vi "testMaster.vi"() -> ()   [LabVIEW 2015]
uses:
  support/Slave Device State.ctl
  support/Network Stream Writer.ctl
  NetworkStream/NetworkStreamData.ctl
  <vilib>/dex/Stream Element Allocation Mode.ctl
  <resource>/objmgr/ni.dex.rc
  NetworkStream/NetworkStream.lvlib
panel:
  out "DeviceState":T1
  in  "data":i32
  in  "Message":string
  in  "stop VI":bool
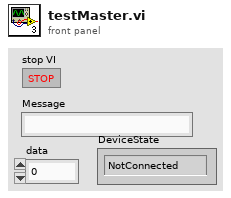
[diagram p1: front panel]
types:
  T1 = typedef "Slave Device State.ctl" = enum16{"NotConnected", "Connected"}
  T2 = typedef "Network Stream Writer.ctl" = cluster{"Hash":u64, "writer endpoint":refnum<k21>, "Sequence Number":u64}
  T3 = typedef "NetworkStream.lvlib/NetworkStreamData.ctl" = cluster{"Command/Status":string, "Data":variant, "Session Hash":u64, "Sequence Number":u64}
  T4 = typedef "Stream Element Allocation Mode.ctl" = u32
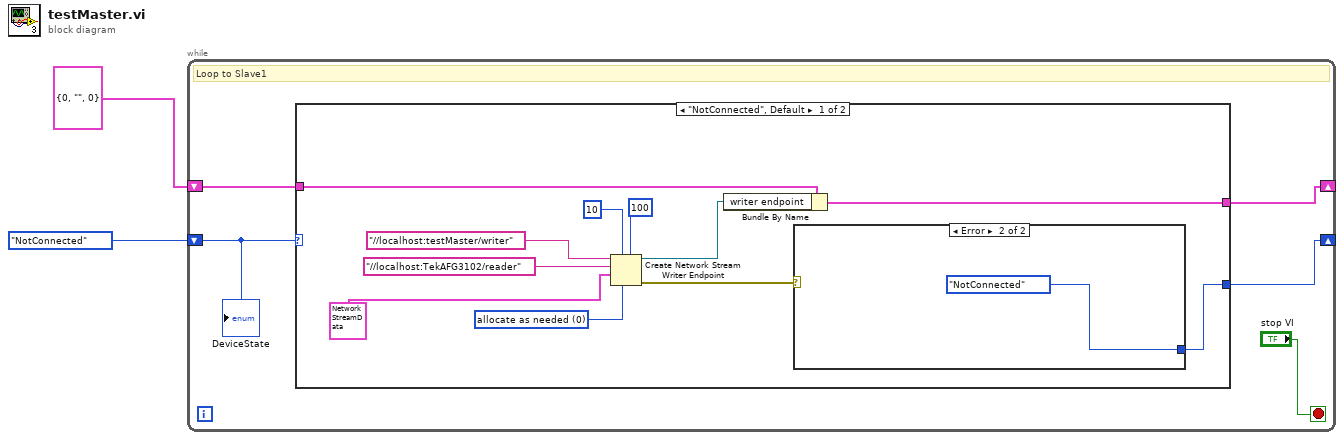
[diagram p0: block diagram]
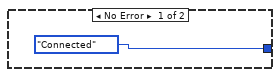
[diagram p2: hidden frame]
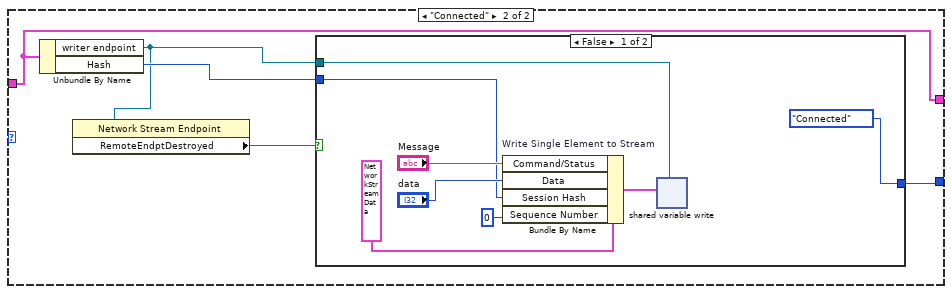
[diagram p3: hidden frame]
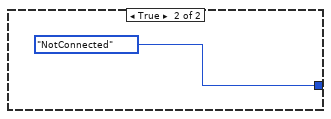
[diagram p4: hidden frame]
diagram:
  n1 = while {
    shift-right: [w5] -> _
    shift-left: T2 {"Hash"=0, "writer endpoint"="", "Sequence Number"=0} ("DeviceData") -> [w6]
    shift-right: [w4] -> _
    shift-left: Slave_Device_State."NotConnected" ("DeviceState") -> [w7]
    stop <- "stop VI" stop-if-true
    # "Loop to Slave1"
    n2 = case shown="\"NotConnected\", Default" w7 {
      tunnel: w6 -> [w18 w24]
      tunnel: [w15 w24] -> w5
      tunnel: [w13 w21] -> w4
      frame "NotConnected", Default {
        w10 = T4 0 items=["allocate as needed", "pre-allocate"] ("element allocation mode")
        n3 = Create Network Stream Writer Endpoint(5:100 ("timeout in ms (-1)"), 6:w10, 7:10 ("writer buffer size"), 9:T3 {"Command/Status"="", "Data"=variant, "Session Hash"=0, "Sequence Number"=0} ("NetworkStreamCluster"), 10:"//localhost:TekAFG3102/reader" ("reader url"), 11:"//localhost:testMaster/writer" ("writer url")) -> (0:w14:errorcluster, 3:w16:refnum<k21>)  [unwired: 1 in]
        n4 = Bundle By Name(cluster=w18, "writer endpoint"=w16) -> (w15:T2)
        n5 = case shown="Error" w14 {
          tunnel: [Slave_Device_State."Connected" ("DeviceState") Slave_Device_State."NotConnected" ("DeviceState")] -> w13
          frame No Error {
          }
          frame Error {
          }
        }
      }
      frame "Connected" {
        n6 = Unbundle By Name(w24) -> ("writer endpoint"=w23:refnum<k21>, "Hash"=w25:u64)
        n7 = property class="Network Stream Endpoint"(reference=w23) -> ("RemoteEndptDestroyed"=w22:bool)  [unwired: 1 in, 2 out]
        n8 = case shown="False" w22 {
          tunnel: w25 -> [w29 _]
          tunnel: w23 -> [w28 _]
          tunnel: [Slave_Device_State."Connected" ("DeviceState") Slave_Device_State."NotConnected" ("DeviceState")] -> w21
          frame False {
            n9 = Bundle By Name(cluster=T3 {"Command/Status"="", "Data"=variant, "Session Hash"=0, "Sequence Number"=0} ("NetworkStreamCluster"), "Command/Status"="Message", "Data"="data", "Session Hash"=w29, "Sequence Number"=u64 0) -> (w27:T3)
            n10 = shared-variable-write "Write Single Element to Stream"(w28, w27) -> ()  [unwired: 2 in, 3 out]
          }
          frame True {
          }
        }
      }
    }
    "DeviceState" <- w7
  }
